vi "ToString.vi"(8 "error in (no error)":errorcluster, 11 "Double D Element in":refnum<class "Double D Element.lvclass">) -> (0 "error out":errorcluster, 2 "String":string, 3 "Double D Element out":refnum<class "Double D Element.lvclass">)   [LabVIEW 2018, in "D Datagrid Library.lvlib" / "Double D Element.lvclass"]
uses:
  Double D Element.lvclass
  Double D Element.lvclass/Double D Element.ctl
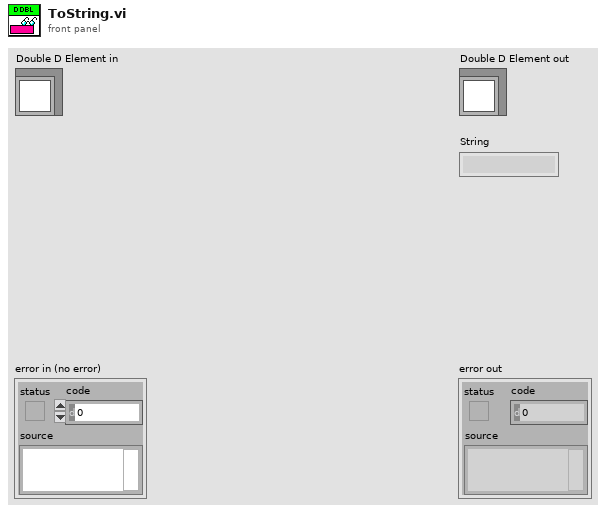
[diagram p1: front panel]
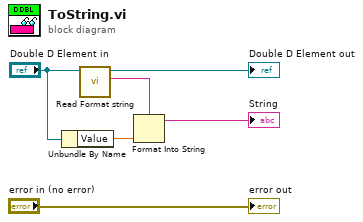
[diagram p0: block diagram]
diagram:
  n1 = Unbundle By Name("Double D Element in") -> ("Value"=w5:dbl)
  n2 = call-dynamic "Read Format string.vi"("Double D Element in"="Double D Element in") -> ("Format string"=w1:string, "Double D Element out"=→"Double D Element out":refnum<class "Double D Element.lvclass">)  [unwired: 8 in, 1 out]
  n3 = Format Into String(format string=w1, w5) -> (resulting string=→"String":string)  [unwired: 2 in, 1 out]
  "error out" <- "error in (no error)"
